vi "op_GetIDs.vi"(9 "list ID file name":string="ID list.txt", 10 "IP address":string="172.16.14.23") -> (0 "error out":errorcluster, 1 "Chip ID list":u32[](array[numeric]) format="%.0x", 2 "Layer ID list (ordered)":u32[](array[numeric]) format="%.0x", 3 "All ID list":u32[](array[numeric]) format="%.0x", 5 "IDs summary":string)   [LabVIEW 2015, in "VIPM2.lvlib"]
doc: "Operation: GetIDs, make summary, save to file."
uses:
  VIPM2.lvlib
panel:
  # "Operation: GetIDs, make summary, save to file"
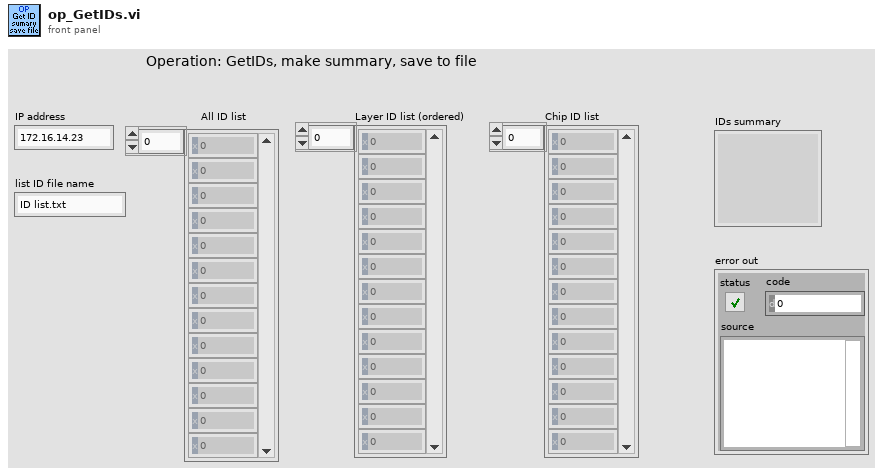
[diagram p1: front panel]
types:
  T1 = enum16{"open", "replace", "create", "open or create", "replace or create", "replace or create with confirmation"}
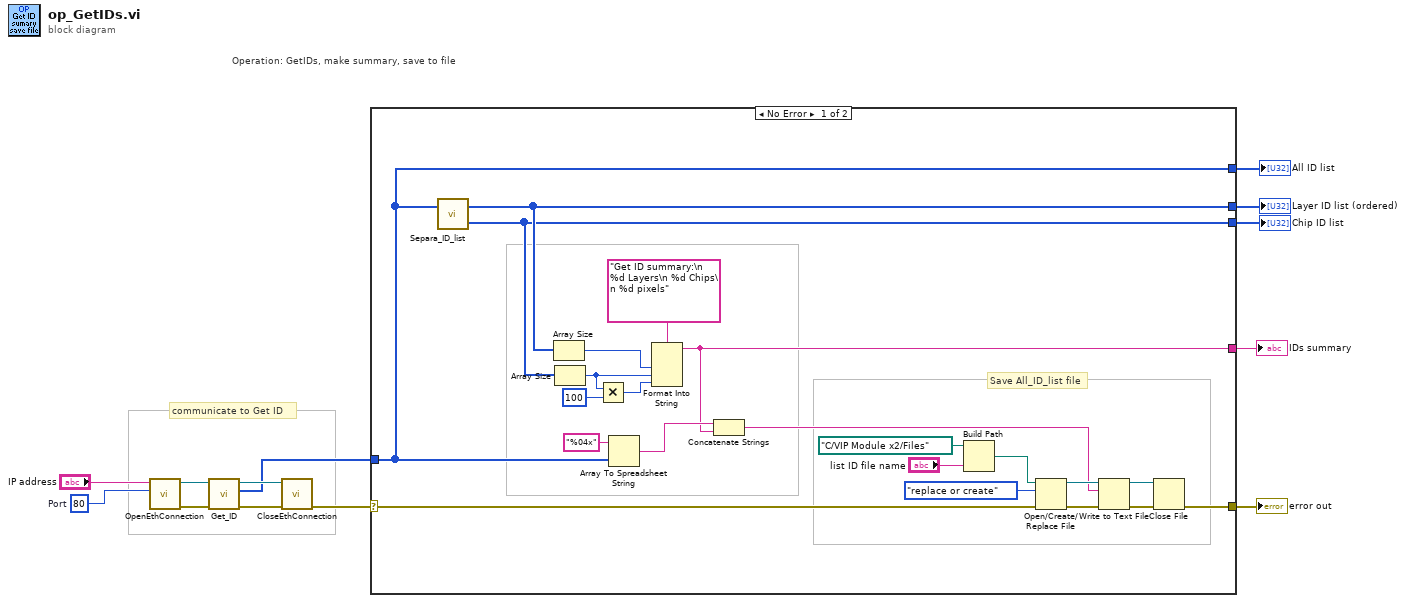
[diagram p0: block diagram]
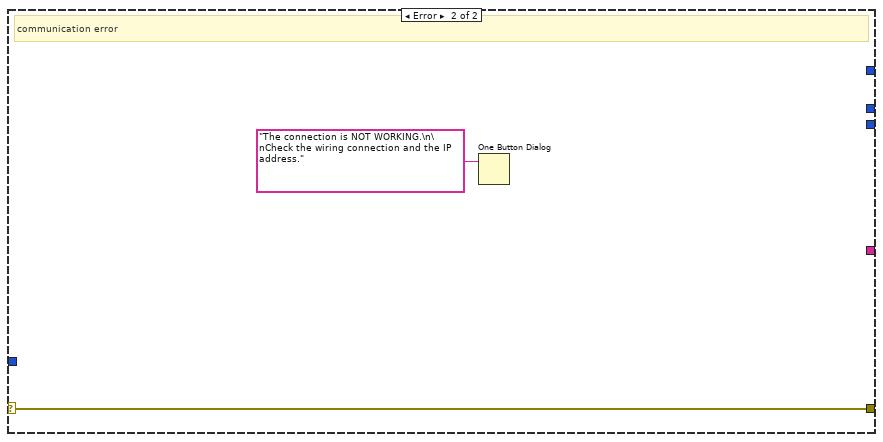
[diagram p2: hidden frame]
diagram:
  w8 = u16 80  # Port
  # "communicate to Get ID"
  # "Operation: GetIDs, make summary, save to file"
  n1 = call "OpenEthConnection.vi"("Port"=w8, "IP address"="IP address") -> ("error out"=w12:errorcluster, "connection ID out"=w13:refnum<k5>)  [unwired: 7 in, 1 out]
  n2 = call "Get_ID.vi"("error in (no error)"=w12, "connection ID"=w13) -> ("error out"=w10:errorcluster, "All ID list"=w5:u32[], "connection ID out"=w11:refnum<k5>)  [unwired: 6 in, 1 out]
  n3 = call "CloseEthConnection.vi"("error in (no error)"=w10, "connection ID"=w11) -> ("error out"=w7:errorcluster)  [unwired: 9 in]
  n4 = case shown="No Error" w7 {
    selector: w7 -> [w23 w37]
    tunnel: [w33 w37] -> w6
    tunnel: w5 -> [w27 _]
    tunnel: [w27 _] -> w4
    tunnel: [w35 _] -> w3
    tunnel: [w34 _] -> w2
    tunnel: [w24 _] -> w1
    frame No Error {
      # "Save All_ID_list file"
      n5 = call "Separa_ID_list.vi"("All ID list"=w27) -> ("Chip ID list"=w34:u32[], "Layer ID list (ordered)"=w35:u32[])  [unwired: 1 in]
      n6 = Array Size(array=w35) -> (size(s)=w29:i32)
      n7 = Array Size(array=w34) -> (size(s)=w31:i32)
      n8 = Multiply(x=w31, y=100) -> (x*y=w30:i32)
      n9 = Array To Spreadsheet String(array=w27, 3:"%04x" ("format string")) -> (spreadsheet string=w25:string)  [unwired: 1 in]
      n10 = Format Into String "Format Into String"(format string="Get ID summary:\n %d Layers\n %d Chips\n %d pixels", w29, w31, w30) -> (resulting string=w24:string)  [unwired: 2 in, 1 out]
      n11 = Concatenate Strings "Concatenate Strings"(w25, w24) -> (w19:string)
      n12 = Build Path(base path=path "C:/VIP Module x2/Files" ("file path (use dialog)"), name or relative path="list ID file name") -> (appended path=w15:path)
      n13 = Open/Create/Replace File ("Create/Replace File")(file path (use dialog)=w15, error in=w23, operation (0:open)=T1."replace or create") -> (refnum out=w20:refnum<file>, error out=w21:errorcluster)  [unwired: 3 in, 1 out]
      n14 = Write to Text File(file (use dialog)=w20, text=w19, error in=w21) -> (refnum out=w17:refnum<file>, error out=w18:errorcluster)  [unwired: 1 in, 1 out]
      n15 = Close File(refnum=w17, error in=w18) -> (error out=w33:errorcluster)  [unwired: 1 out]
    }
    frame Error {
      # "communication error"
      n16 = One Button Dialog(message="The connection is NOT WORKING.\n\nCheck the wiring connection and the IP address.") -> ()  [unwired: 1 in, 1 out]
    }
  }
  "error out" <- w6
  "All ID list" <- w4
  "Layer ID list (ordered)" <- w3
  "Chip ID list" <- w2
  "IDs summary" <- w1
